vi "write_timestamp_to_file.vi"(8 "clock freq":i64, 9 "index":i32, 10 "metadata":i64, 11 "free run save path":path) -> ()   [LabVIEW 2019]
panel:
  out "MetaData 3":i64
  out "MetaData 2":i64
  out "MetaData":i64
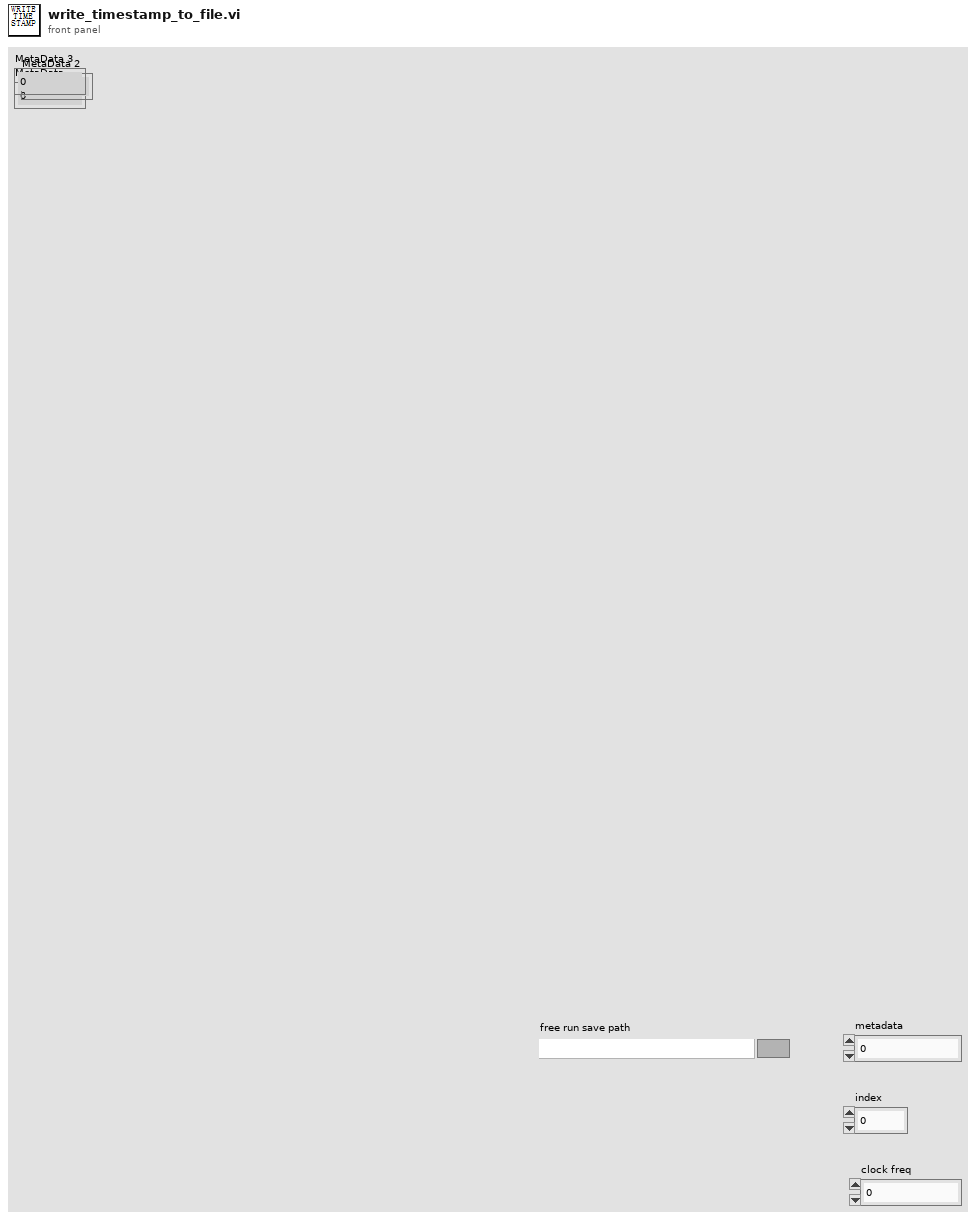
[diagram p1: front panel]
types:
  T1 = enum16{"open", "replace", "create", "open or create", "replace or create", "replace or create with confirmation"}
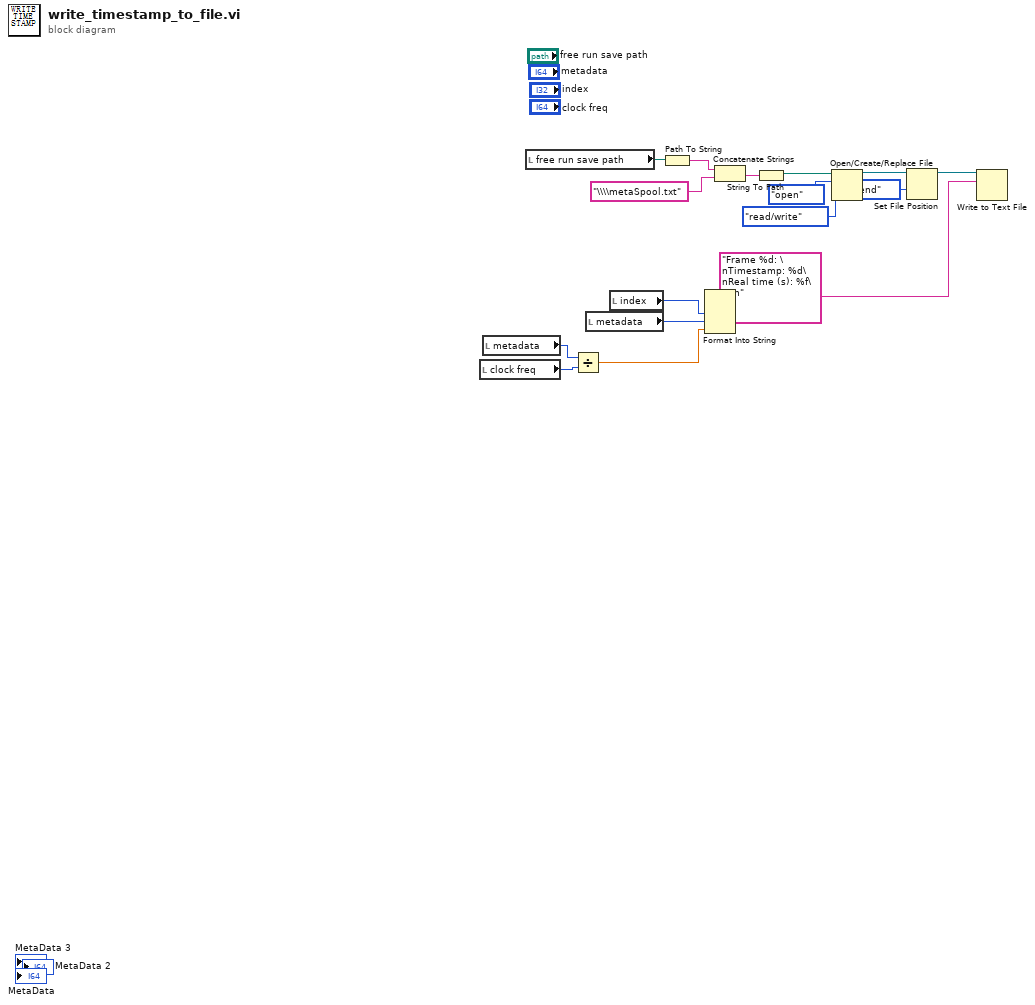
[diagram p0: block diagram]
diagram:
  n1 = local read "clock freq"() -> (w2:i64)
  n2 = local read "metadata"() -> (w3:i64)
  n3 = local read "free run save path"() -> (w17:path)
  n4 = Divide(x=w3, y=w2) -> (x/y=w1:dbl)
  n5 = local read "metadata"() -> (w5:i64)
  n6 = local read "index"() -> (w6:i32)
  n7 = Path To String(path=w17) -> (string=w15:string)
  n8 = Format Into String(format string="Frame %d: \nTimestamp: %d\nReal time (s): %f\n\\n", w6, w5, w1) -> (resulting string=w7:string)  [unwired: 2 in, 1 out]
  n9 = Concatenate Strings(w15, "\\\\metaSpool.txt" ("format string")) -> (w14:string)
  n10 = String To Path(string=w14) -> (path=w13:path)
  n11 = Open/Create/Replace File(file path (use dialog)=w13, operation (0:open)=T1."open", access (0:read/write)=enum16{"read/write", "read-only", "write-only"}."read/write") -> (refnum out=w10:refnum<file>)  [unwired: 3 in, 2 out]
  n12 = Set File Position(refnum=w10, from (0:start)=enum16{"start", "end", "current"}."end") -> (refnum out=w8:refnum<file>)  [unwired: 2 in, 1 out]
  n13 = Write to Text File(file (use dialog)=w8, text=w7) -> ()  [unwired: 2 in, 3 out]
